vi "Get MenuItem Properties.vi"(0 "NotifyIcon in":refnum<class "NotifyIcon.lvclass">, 5 "MenuItem":refnum<k24>, 11 "error in (no error)":errorcluster) -> (4 "dub NotifyIcon":refnum<class "NotifyIcon.lvclass">, 6 "MenuItem out":refnum<k24>, 10 "MenuItem Properties":T1, 15 "error out":errorcluster)   [LabVIEW 2017, in "NotifyIcon.lvclass"]
doc: "This VI gets the properties for the MenuItem referenced by the <b>MenuItem</b> input.\n\n\nStinus Olsen\nCIM Industrial Systems A/S\n22. Feb. 2011 15:04\nmailto: seo@cim.as"
uses:
  NotifyIcon.lvclass
  System.Windows.Forms
  Controls/MenuItem Properties.ctl
panel:
  # "This VI belongs to the NotifyIcon Toolset. \nA toolset that makes it easy to create, control and manipulate a notification icon in the notification area of the Windows taskbar.\nThe toolset requires Microsoft .NET framework 2.0\n\n\nNOTICE -- YOU MUST LEAVE THIS NOTICE IN PLACE.  PER THE TERMS OF THE LICENSE BELOW, YOU MAY SUBLICENSE THIS SOFTWARE \nIN ANY WAY THAT DOES NOT CONFLICT WITH THIS LICENSE.\n\n### BSD License (http://www.opensource.org/licenses/bsd-license.php) Begin ###\n \nCopyright (c) 2011, Stinus Olsen <seo@cim.as>\n\nAll rights reserved.\n\nRedistribution and use in source and binary forms, with or without modification, are permitted provided that the following conditions are met:\n\n    * Redistributions of source code must retain the above copyright notice, this list of conditions and the following disclaimer.\n    * Redistributions in binary form must reproduce the above copyright notice, this list of conditions and the following disclaimer in the \n       documentation and/or other materials provided with the distribution.\n    * Neither the name of CIM Industrial Systems nor the names of its contributors may be used to endorse or promote products derived \n       from this software without specific prior written permission.\n\nTHIS SOFTWARE IS PROVIDED BY THE COPYRIGHT HOLDERS AND CONTRIBUTORS \"AS IS\" AND ANY EXPRESS OR IMPLIED WARRANTIES, \nINCLUDING, BUT NOT LIMITED TO, THE IMPLIED WARRANTIES OF MERCHANTABILITY AND FITNESS FOR A PARTICULAR PURPOSE ARE \nDISCLAIMED. IN NO EVENT SHALL THE COPYRIGHT OWNER OR CONTRIBUTORS BE LIABLE FOR ANY DIRECT, INDIRECT, INCIDENTAL,\n SPECIAL, EXEMPLARY, OR CONSEQUENTIAL DAMAGES (INCLUDING, BUT NOT LIMITED TO, PROCUREMENT OF SUBSTITUTE GOODS OR \nSERVICES; LOSS OF USE, DATA, OR PROFITS; OR BUSINESS INTERRUPTION) HOWEVER CAUSED AND ON ANY THEORY OF LIABILITY, \nWHETHER IN CONTRACT, STRICT LIABILITY, OR TORT (INCLUDING NEGLIGENCE OR OTHERWISE) ARISING IN ANY WAY OUT OF THE USE \nOF THIS SOFTWARE, EVEN IF ADVISED OF THE POSSIBILITY OF SUCH DAMAGE.\n\n### BSD License End ###"
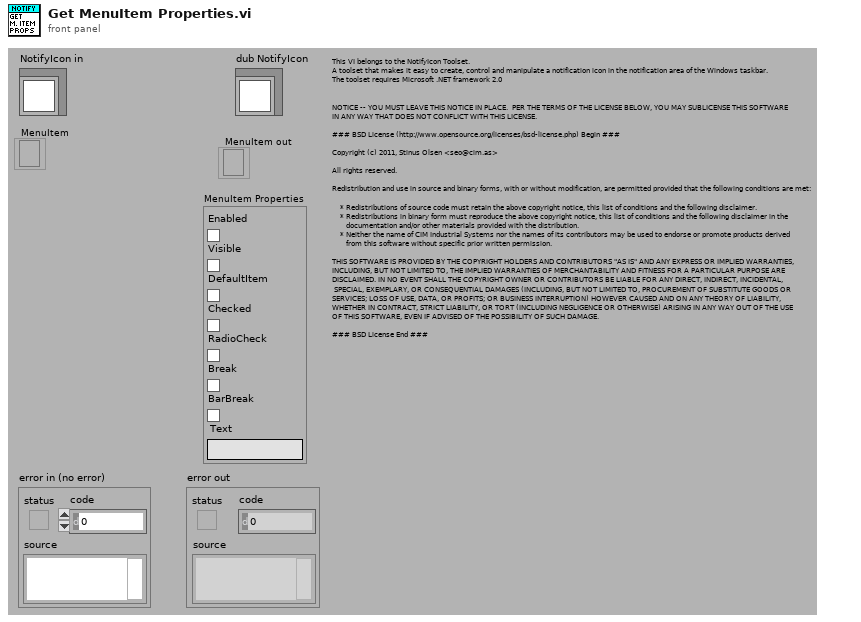
[diagram p1: front panel]
types:
  T1 = typedef "NotifyIcon.lvclass/MenuItem Properties.ctl" = cluster{"Enabled":bool, "Visible":bool, "DefaultItem":bool, "Checked":bool, "RadioCheck":bool, "Break":bool, "BarBreak":bool, "Text":string}
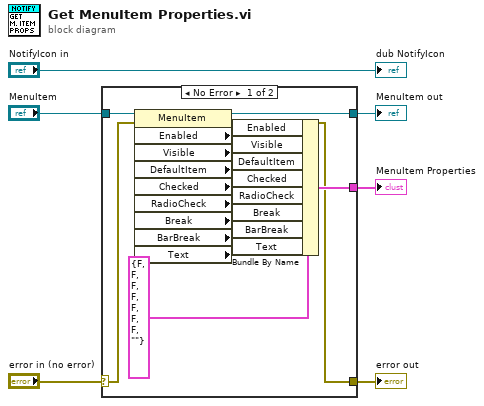
[diagram p0: block diagram]
diagram:
  n1 = case shown="No Error" "error in (no error)" {
    selector: "error in (no error)" -> [w19 w22]
    tunnel: [w8 w22] -> w5
    tunnel: "MenuItem" -> [w20 w21]
    tunnel: [w9 _] -> w2
    tunnel: [w7 w21] -> w1
    frame No Error {
      n2 = property class="MenuItem"(reference=w20, error in=w19) -> (reference out=w7:refnum<k24>, error out=w8:errorcluster, "Enabled"=w17:bool, "Visible"=w16:bool, "DefaultItem"=w15:bool, "Checked"=w14:bool, "RadioCheck"=w13:bool, "Break"=w12:bool, "BarBreak"=w11:bool, "Text"=w10:string)
      n3 = Bundle By Name(cluster=T1 {"Enabled"=FALSE, "Visible"=FALSE, "DefaultItem"=FALSE, "Checked"=FALSE, "RadioCheck"=FALSE, "Break"=FALSE, "BarBreak"=FALSE, "Text"=""} ("MenuItem Properties"), "Enabled"=w17, "Visible"=w16, "DefaultItem"=w15, "Checked"=w14, "RadioCheck"=w13, "Break"=w12, "BarBreak"=w11, "Text"=w10) -> (w9:T1)
    }
    frame Error {
    }
  }
  "error out" <- w5
  "MenuItem Properties" <- w2
  "MenuItem out" <- w1
  "dub NotifyIcon" <- "NotifyIcon in"
